vi "histogram2_cam.vi"() -> ()   [LabVIEW 2020]
uses:
  <vilib>/userdefined/High Color/IMAQdx.ctl
  <vilib>/vision/driver/NI_Vision_Acquisition_Software.lvlib
  <vilib>/vision/NI_Vision_Development_Module.lvlib
panel:
  out "(hi.lo)":u32(colorbox)
  out "색상":T1(ring)
  out "색숫자":u32
  out "히스토그램2":u8[][](graph)
  out "Image Out":T2(plugin-control)
  in  "캡쳐":bool
  in  "정지":bool
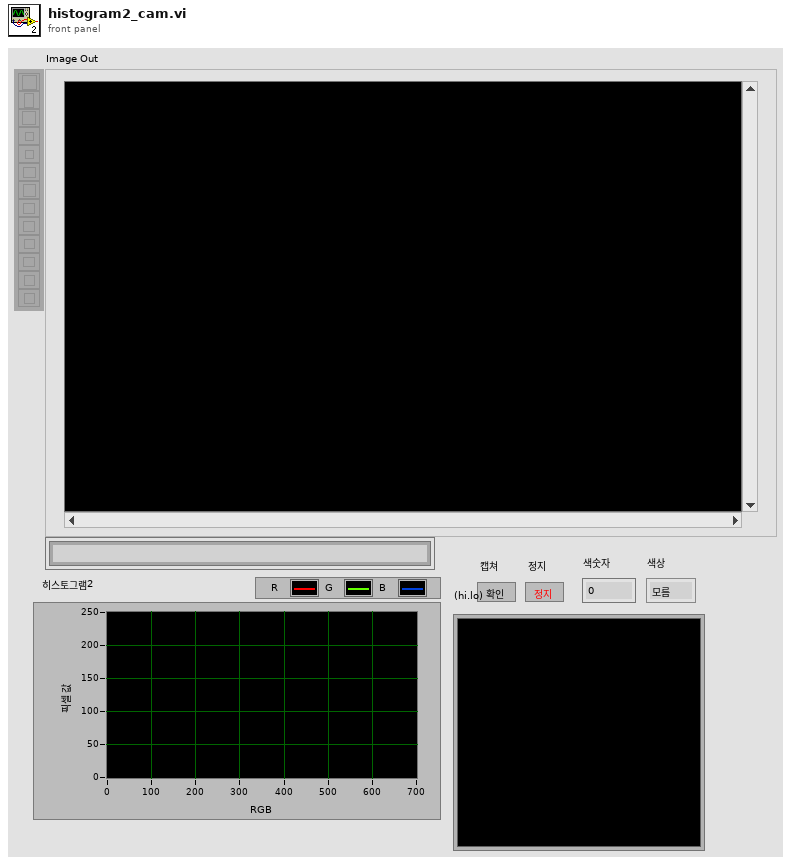
[diagram p1: front panel]
types:
  T1 = enum16{"모름", "빨강", "녹색", "노랑", "파랑", "보라", "하늘", "흰색"}
  T2 = typedef "IMAQ Image.ctl" = refnum<image>
  T3 = typedef "IMAQdx.ctl" = refnum<k21>
  T4 = enum16{"모름", "빨강", "녹색", "노랑", "파랑", "보라", "하늘", "흰색"}[]
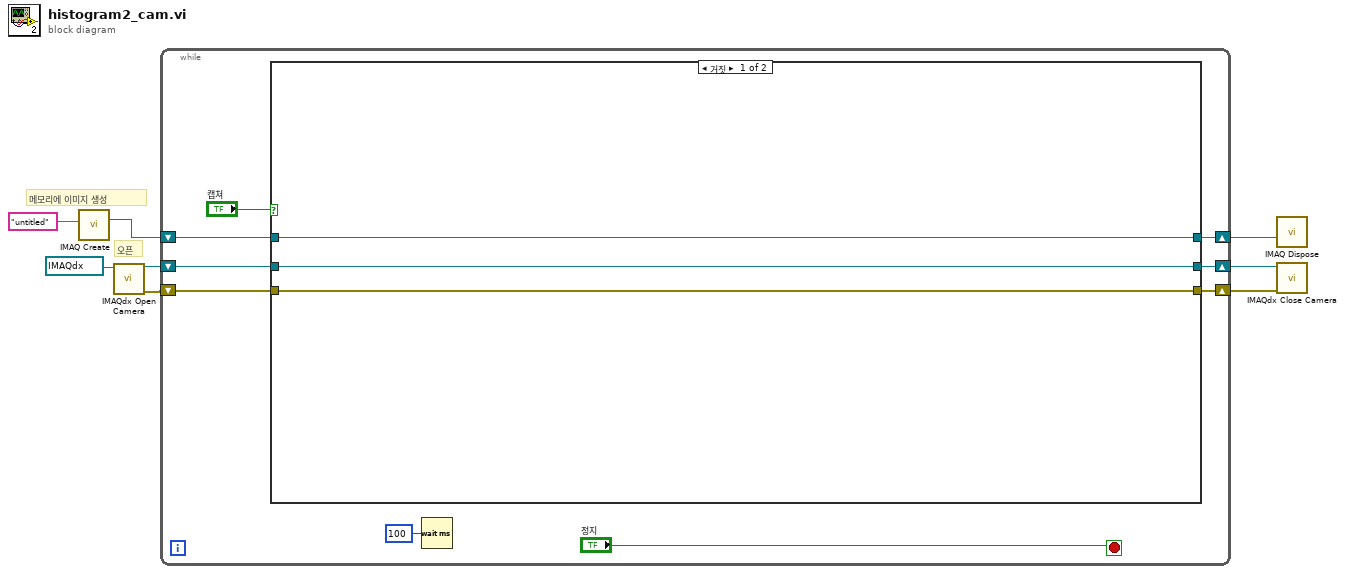
[diagram p0: block diagram]
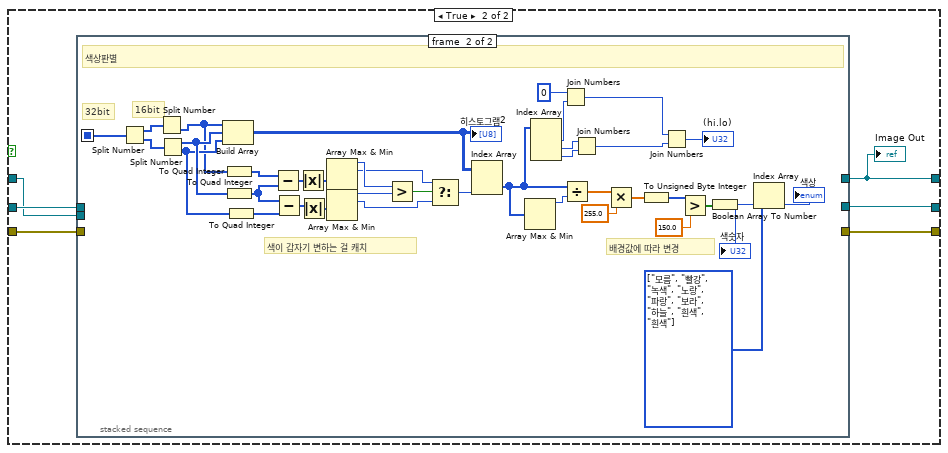
[diagram p2: hidden frame]
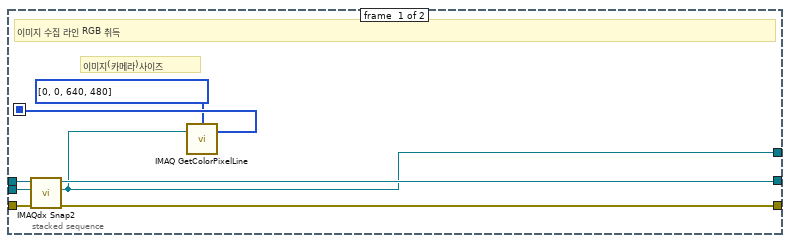
[diagram p3: hidden frame]
diagram:
  # "오픈"
  # "메모리에 이미지 생성"
  n1 = call "IMAQ Create"("Image Name"="untitled") -> ("New Image"=w6:T2)  [unwired: 4 in, 1 out]
  n2 = call <vilib>:"IMAQdx Open Camera.vi"("Session In"=T3 "cam0") -> ("error out"=w5:errorcluster, "Session Out"=w7:T3)  [unwired: 9 in]
  n3 = while {
    shift-right: [w15] -> w4
    shift-left: w7 -> [w17]
    shift-right: [w13] -> w1
    shift-left: w6 -> [w16]
    shift-right: [w14] -> w3
    shift-left: w5 -> [w9]
    stop <- "정지" stop-if-true
    n4 = case shown="거짓" "캡쳐" {
      tunnel: w17 -> [w19 w26]
      tunnel: w16 -> [w20 w25]
      tunnel: w9 -> [w18 w24]
      tunnel: [w19 w23] -> w15
      tunnel: [w18 w22] -> w14
      tunnel: [w20 w21] -> w13
      frame False {
      }
      frame True {
        n5 = stacked-sequence {
          seq-local: [w29 _] -> [_ w72]
          tunnel: w26 -> [w34 _]
          tunnel: w25 -> [w33 _]
          tunnel: w24 -> [w32 _]
          tunnel: [w31 _] -> w23
          tunnel: [w30 _] -> w22
          tunnel: [w27 _] -> w21
          frame #0 {
            # "이미지(카메라)사이즈"
            # "이미지 수집 라인 RGB 취득"
            n6 = call <vilib>:"IMAQdx Snap2.vi"("error in"=w32, "Image In"=w33, "Session In"=w34) -> ("error out"=w30:errorcluster, "Image Out"=w27:T2, "Session Out"=w31:T3)  [unwired: 6 in]
            n7 = call "IMAQ GetColorPixelLine"("Line Coordinates"=i32[] [0, 0, 640, 480], "Image"=w27) -> ("Pixels Line (U32)"=w29:u32[])  [unwired: 2 in, 2 out]
          }
          frame #1 {
            w44 = T4 [enum."모름", enum."빨강", enum."녹색", enum."노랑", enum."파랑", enum."보라", enum."하늘", enum."흰색", enum."흰색"] items=["모름", "빨강", "녹색", "노랑", "파랑", "보라", "하늘", "흰색"] ("배열")
            # "배경값에 따라 변경"
            # "색이 갑자기 변하는 걸 캐치"
            # "16bit"
            # "32bit"
            # "색상판별"
            n8 = Split Number(x=w72) -> (hi(x)=w71:u16[], lo(x)=w70:u16[])
            n9 = Split Number(x=w71) -> (lo(x)=w67:u8[])  [unwired: 1 out]
            n10 = Split Number(x=w70) -> (hi(x)=w69:u8[], lo(x)=w68:u8[])
            n11 = Build Array(w67, w69, w68) -> (w58:u8[][])
            "히스토그램2" <- w58
            n12 = To Quad Integer(1:w67) -> (0:w66:i64[])
            n13 = To Quad Integer(1:w69) -> (0:w65:i64[])
            n14 = To Quad Integer(1:w68) -> (0:w64:i64[])
            n15 = Subtract(x=w66, y=w65) -> (x-y=w56:i64[])
            n16 = Subtract(x=w65, y=w64) -> (x-y=w55:i64[])
            n17 = Absolute Value(x=w56) -> (abs(x)=w54:i64[])
            n18 = Absolute Value(x=w55) -> (abs(x)=w53:i64[])
            n19 = Array Max & Min(array=w54) -> (max value=w63:i64, max index (indices)=w60:i32)  [unwired: 2 out]
            n20 = Array Max & Min(array=w53) -> (max value=w62:i64, max index (indices)=w59:i32)  [unwired: 2 out]
            n21 = Greater?(x=w63, y=w62) -> (0:w61:bool)
            n22 = Select(t=w60, s=w61, f=w59) -> (s? t:f=w57:i32)
            n23 = Index Array(array=w58, index (col)=w57) -> (element=w39:u8[])  [unwired: 1 in]
            n24 = Array Max & Min(array=w39) -> (max value=w52:u8)  [unwired: 3 out]
            n25 = Index Array(array=w39) -> (element #1=w38:u8, element #2=w37:u8, element #3=w36:u8)  [unwired: 3 in]
            n26 = Join Numbers(hi=u8 0, lo=w38) -> ((hi.lo)=w42:u16)
            n27 = Divide(x=w39, y=w52) -> (x/y=w51:dbl[])
            n28 = Join Numbers(hi=w37, lo=w36) -> ((hi.lo)=w40:u16)
            n29 = Multiply(x=w51, y=255.0) -> (x*y=w49:dbl[])
            n30 = To Unsigned Byte Integer(number=w49) -> (unsigned 8bit integer=w48:u8[])
            n31 = Join Numbers(hi=w42, lo=w40) -> ((hi.lo)=→"(hi.lo)":u32)
            n32 = Greater?(x=w48, y=150.0) -> (0:w46:bool[])
            n33 = Boolean Array To Number(Boolean array=w46) -> (number=w45:u32)
            "색숫자" <- w45
            n34 = Index Array(array=w44, index=w45) -> (element=→"색상":T1)
          }
        }
        "Image Out" <- w21
      }
    }
    n35 = Wait (ms)(milliseconds to wait=u32 100 ("대기 시간 (ms)")) -> ()  [unwired: 1 out]
  }
  n36 = call "IMAQ Dispose"("Image"=w1) -> ()  [unwired: 5 in, 1 out]
  n37 = call <vilib>:"IMAQdx Close Camera.vi"("error in"=w3, "Session In"=w4) -> ()  [unwired: 9 in, 1 out]
